vi "teater2.vi"() -> ()   [LabVIEW 2013]
uses:
  <vilib>/Platform/TimedLoop/XDataNode/timing_clust.ctl
  <vilib>/Platform/TimedLoop/XDataNode/nitl_modes.ctl
  <vilib>/Platform/TimedLoop/XDataNode/wakeup.ctl
  Controls/DRAM mem type.ctl
  <vilib>/rvi/Emulation/niFpgaSctlEmulationGetInTimedLoop.vi
  <vilib>/rvi/Emulation/niFpgaEmulationReportErrorSimple.vi
  <vilib>/rvi/Emulation/niFpgaGetClockAttributes.vi
  <vilib>/rvi/Emulation/niFpgaCriticalErrorInLSC.vi
  <vilib>/rvi/eio/common/nirviEmuTemplateMethod_errors.vi
  <vilib>/rvi/DataTransferAndStorage/Container/Common/niFpgaContainerGetUniqueNameForEmu.vi
  <vilib>/rvi/Memory/Memory_Emulation/niFpgaMemoryEmulationReadFromVariant.vi
  <vilib>/rvi/Memory/Memory_Emulation/niFpgaMemoryEmulationWriteToVariant.vi
  <vilib>/rvi/Memory/Memory_Emulation/niFpgaMemoryFastEmulationDramWriteAndRequestData.vi
  <vilib>/rvi/Memory/Memory_Emulation/niFpgaMemoryEmulationDramWriteAndRequestData.vi
  <vilib>/Platform/TimedLoop/XDataNode/XDataNode.xnode
  <vilib>/eio/EIONode/EIONode.xnode
  <vilib>/rvi/DataTransferAndStorage/Container/XNode/niFpgaContainer.xnode
  <vilib>/rvi/Memory/Memory_Emulation/niFpgaMemoryEmulationDramRetrieveData.vi
  <vilib>/Platform/TimedLoop/XDataNode/XDNodeRunTimeDep.lvlib
panel:
  out "Missed ret.":u16
  out "missed req.":u16
  in  "Start Add Rd":u16
  in  "Start Add Wr":u16
  out "DRAM Bank 0\\Read_Data_Lower":u16
  out "max(x,y)":u64
  in  "Start read mem":bool
  in  "Start fill mem":bool
  in  "Mem size":u16
  out "AI0":i16
  out "AI1":i16
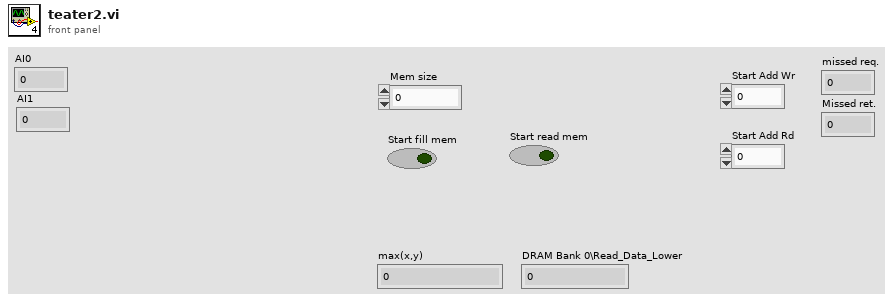
[diagram p1: front panel]
types:
  T1 = typedef "XDNodeRunTimeDep.lvlib/timing_clust.ctl" = cluster{"Expected End [f-1]":u64, "Actual End [f-1]":u64, "Finished Late? [f-1]":bool, "Expected End [i-1]":u64, "Actual End [i-1]":u64, "Finished Late? [i-1]":bool, "Expected Start [i]":u64, "Actual Start [i]":u64, "Expected Start [f]":u64, "Actual Start [f]":u64, "Source Name":string, "Structure Name":string, "Period":i64, "Deadline":i64, "Offset":i64, "Start":i64, "Priority":i32, "Timeout":i32, "Mode":T2, "Wakeup Reason":T3, "Error":errorcluster, "Source Type":string, "Secondary Source Type":string, "Global End Time":u64, "Global Start Time":u64, "Frame Duration":u64, "Iteration Duration":u64, "Assigned CPU":i32, "I/O Scan Engine Mode":u32}
  T2 = typedef "XDNodeRunTimeDep.lvlib/nitl_modes.ctl" = enum32{"No Change", "Process missed periods, maintain original phase", "Discard missed periods, maintain original phase", "Process missed periods, ignore original phase", "Discard missed periods, ignore original phase"}
  T3 = typedef "XDNodeRunTimeDep.lvlib/wakeup.ctl" = enum32{"Normal", "Aborted", "Asynchronous wakeup", "Timing source error", "Timed loop error", "Timeout"}
  T4 = typedef "DRAM mem type.ctl" = cluster{"Low":u64, "High":u64}
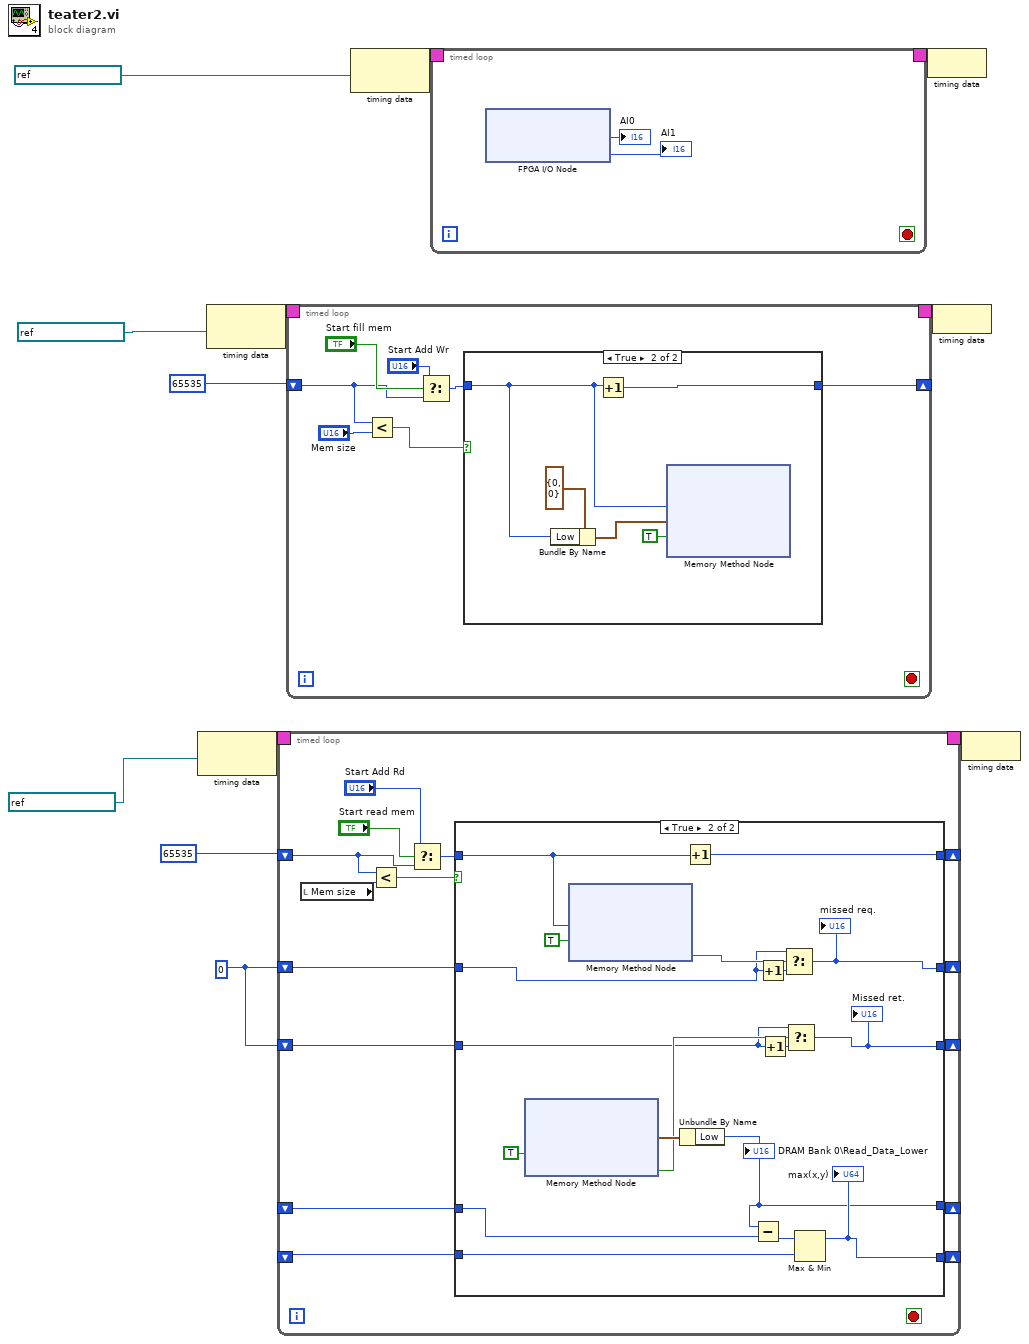
[diagram p0: block diagram]
diagram:
  w1 = u16 0
  n1 = node-c288(refnum<k21> "200 MHz Clock" ("Source Name")) -> (w5:T1)
  n2 = node-c288(refnum<k21> "200 MHz Clock" ("Source Name")) -> (w9:T1)
  n3 = timed-loop {
    timing: w5 -> [_]
    timing-out: [_] -> w4
    shift-right: [w27] -> _
    shift-left: u16 65535 -> [w24]
    shift-right: [w21] -> _
    shift-left: _ -> [w20]
    shift-right: [w19] -> _
    shift-left: _ -> [w18]
    shift-right: [w15] -> _
    shift-left: w1 -> [w16]
    shift-right: [w13] -> _
    shift-left: w1 -> [w14]
    stop <- _ stop-if-true
    n4 = local read "Mem size"() -> (w22:u16)
    n5 = Less?(x=w24, y=w22) -> (x < y?=w26:bool)
    n6 = Select(t="Start Add Rd", s="Start read mem", f=w24) -> (s? t:f=w23:u16)
    n7 = case shown="True" w26 {
      tunnel: w23 -> [w28 w41]
      tunnel: [w28 w46] -> w27
      tunnel: [_ w38] -> w21
      tunnel: w20 -> [_ w45]
      tunnel: [_ w43] -> w19
      tunnel: w18 -> [_ w42]
      tunnel: w16 -> [_ w34]
      tunnel: [_ w35] -> w15
      tunnel: w14 -> [_ w30]
      tunnel: [_ w29] -> w13
      frame False {
      }
      frame True {
        n8 = xnode ("Memory Method Node")("Ready For Output"=TRUE) -> ("Data"=w39:cluster{"Low":u64, "High":u64}, "Output Valid"=w31:bool)  [unwired: 1 in, 1 out]
        n9 = xnode ("Memory Method Node")("Address"=w41, "Input Valid"=TRUE) -> ("Ready For Input"=w36:bool)  [unwired: 1 in, 1 out]
        n10 = Unbundle By Name(w39) -> ("Low"=w38:u64)
        "DRAM Bank 0\\Read_Data_Lower" <- w38
        n11 = Increment(x=w41) -> (x+1=w46:u16)
        n12 = Subtract(x=w38, y=w45) -> (x-y=w44:u64)
        n13 = Increment(x=w34) -> (x+1=w33:u16)
        n14 = Increment(x=w30) -> (x+1=w32:u16)
        n15 = Select(t=w34, s=w36, f=w33) -> (s? t:f=w35:u16)
        "missed req." <- w35
        n16 = Select(t=w30, s=w31, f=w32) -> (s? t:f=w29:u16)
        "Missed ret." <- w29
        n17 = Max & Min(x=w44, y=w42) -> (max(x,y)=w43:u64)  [unwired: 1 out]
        "max(x,y)" <- w43
      }
    }
  }
  n18 = timed-loop {
    timing: w9 -> [_]
    timing-out: [_] -> w8
    shift-right: [w54] -> _
    shift-left: u16 65535 -> [w51]
    stop <- _ stop-if-true
    n19 = Less?(x=w51, y="Mem size") -> (x < y?=w53:bool)
    n20 = Select(t="Start Add Wr", s="Start fill mem", f=w51) -> (s? t:f=w50:u16)
    n21 = case shown="True" w53 {
      tunnel: w50 -> [w56 w58]
      tunnel: [w56 w61] -> w54
      frame False {
      }
      frame True {
        n22 = Bundle By Name(cluster=T4 {"Low"=0, "High"=0}, "Low"=w58) -> (w57:T4)
        n23 = Increment(x=w58) -> (x+1=w61:u16)
        n24 = xnode ("Memory Method Node")("Address"=w58, "Data"=w57, "Input Valid"=TRUE) -> ()  [unwired: 1 in, 2 out]
      }
    }
  }
  n25 = node-c288(refnum<k21> "100 MHz Clock" ("Source Name")) -> (w12:T1)
  n26 = timed-loop {
    timing: w12 -> [_]
    timing-out: [_] -> w11
    stop <- _ stop-if-true
    n27 = xnode "FPGA I/O Node"() -> ("IO Module\\AI 0"=→"AI0":i16, "IO Module\\AI 1"=→"AI1":i16)  [unwired: 2 in, 2 out]
  }
  n28 = node-c288(w11) -> ()
  n29 = node-c288(w8) -> ()
  n30 = node-c288(w4) -> ()
